vi "Write Master_Slave.vi"(8 "error in (no error)":errorcluster, 10 "Master/Slave":enum32{"Master", "Slave"}(ring), 11 "Set Master or Slave Msg in":refnum<class "Set Master or Slave Msg.lvclass">) -> (0 "error out":errorcluster, 3 "Set Master or Slave Msg out":refnum<class "Set Master or Slave Msg.lvclass">)   [LabVIEW 2016, in "Controller UI.lvlib" / "Set Master or Slave Msg.lvclass"]
uses:
  <userlib>/Common Components/Controller UI Messages/Set Master or Slave Msg/Set Master or Slave Msg.lvclass
  <userlib>/Common Components/Controller UI Messages/Set Master or Slave Msg/Set Master or Slave Msg.lvclass/Set Master or Slave Msg.ctl
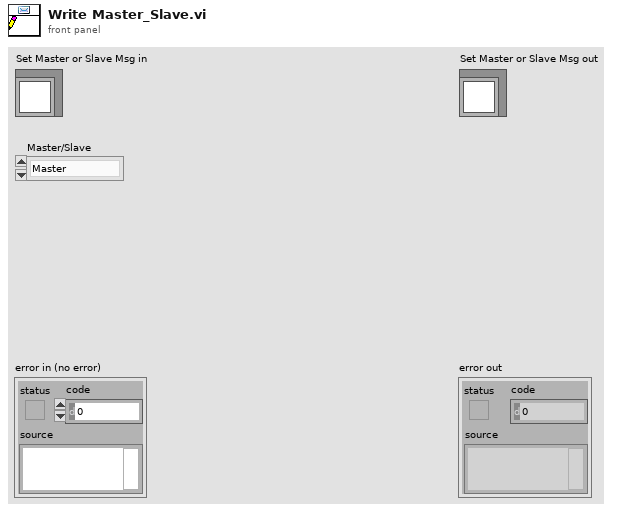
[diagram p1: front panel]
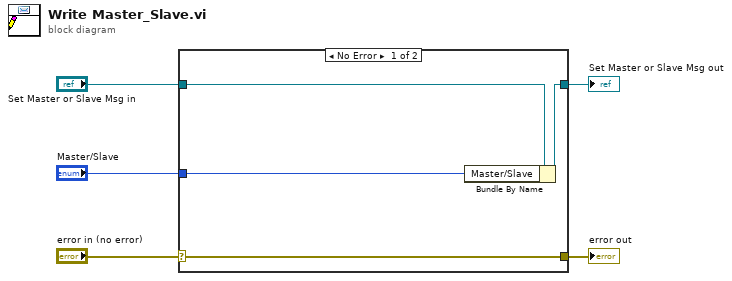
[diagram p0: block diagram]
diagram:
  n1 = case shown="No Error" "error in (no error)" {
    selector: "error in (no error)" -> [w9 w10]
    tunnel: [w9 w10] -> w4
    tunnel: [w7 w11] -> w2
    tunnel: "Set Master or Slave Msg in" -> [w8 w11]
    tunnel: "Master/Slave" -> [w6 _]
    frame No Error {
      n2 = Bundle By Name(cluster=w8, "Master/Slave"=w6) -> (w7:refnum<class "Set Master or Slave Msg.lvclass">)
    }
    frame Error {
    }
  }
  "error out" <- w4
  "Set Master or Slave Msg out" <- w2
